vi "Prompt for File Path.vi"(0 "reference in":refnum<class "Generic Utilities.lvclass">, 5 "error in (no error)":errorcluster, 7 "Start Path":path, 9 "File Type":T1(ring)) -> (13 "selected path":path, 14 "reference out":refnum<class "Generic Utilities.lvclass">, 19 "error out":errorcluster)   [LabVIEW 2020, in "Generic Utilities.lvclass"]
uses:
  Generic Utilities.lvclass
  <vilib>/Utility/sysdir.llb/System Directory Type.ctl
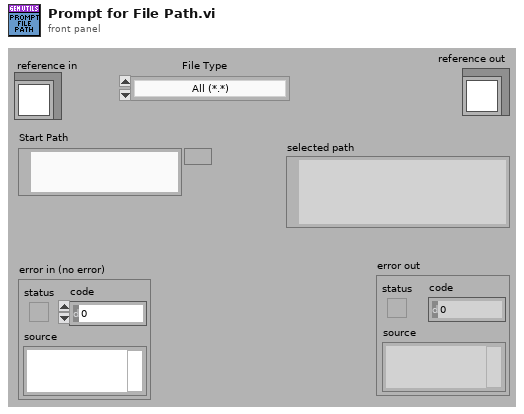
[diagram p1: front panel]
types:
  T1 = enum16{"All (*.*)", "Text (*.txt)", "Word (*.doc)", "Excel (*.xls)"}
  T2 = typedef "Generic Utilities.lvclass/ObjectAttributes.ctl" = cluster{"GUI Parameters":T3, "State Machine Control":cluster{"Timeout":i32, "State Queue":string[], "State History":string[], "State History Length":i32}, "Logging File Path":path, "OBJ not a refnum?":bool, "Timer Start":timestamp, "FP Refnums":T4}
  T3 = typedef "Generic Utilities.lvclass/GUI Parameters.ctl" = cluster{"Application Name":string, "GUI VI Ref":refnum<vi>, "Close Panel?":bool, "Message Window ref":refnum<vi>, "Version #":string}
  T4 = typedef "Generic Utilities.lvclass/FP Refnums.ctl" = cluster{"Panel refnum":refnum<vi>, "Control Labels":string[], "Refnums":refnum<vi>[]}
  T5 = typedef "System Directory Type.ctl" = i32
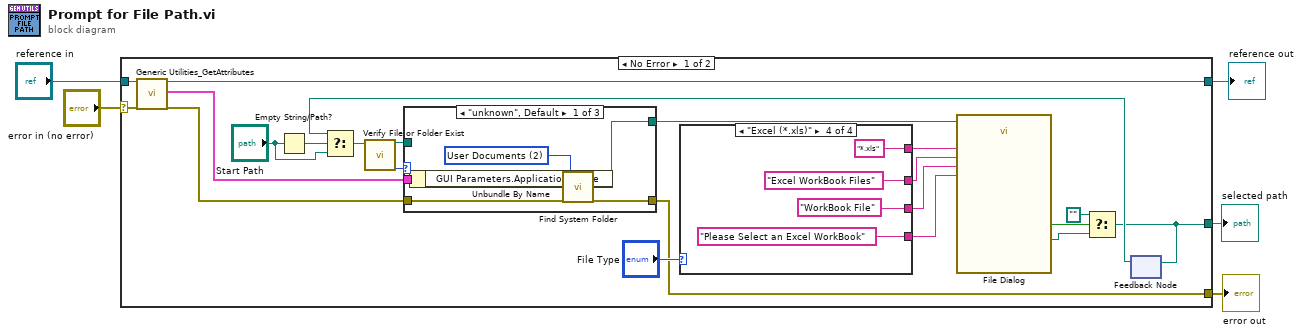
[diagram p0: block diagram]
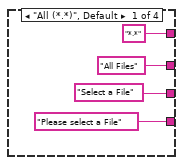
[diagram p2: hidden frame]
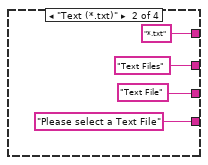
[diagram p3: hidden frame]
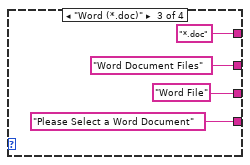
[diagram p4: hidden frame]
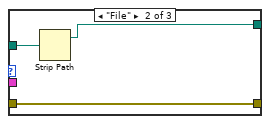
[diagram p5: hidden frame]
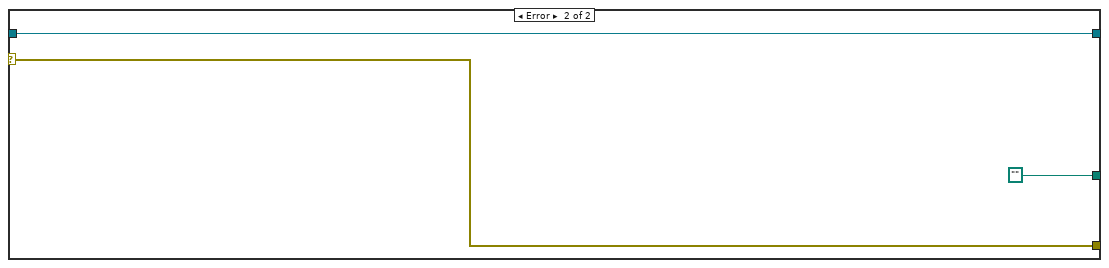
[diagram p7: hidden frame]
diagram:
  n1 = case shown="No Error" "error in (no error)" {
    selector: "error in (no error)" -> [w27 w57]
    tunnel: [w11 w57] -> w4
    tunnel: [w26 w56] -> w2
    tunnel: "reference in" -> [w24 w56]
    tunnel: [w7 path ""] -> w1
    frame No Error {
      n2 = call "Generic Utilities_GetAttributes.vi"("reference in"=w24, "error in (no error)"=w27) -> ("reference out"=w26:refnum<class "Generic Utilities.lvclass">, "attributes"=w25:T2, "error out"=w23:errorcluster)  [unwired: 14 in, 1 out]
      n3 = Empty String/Path?(string/path="Start Path") -> (empty?=w9:bool)
      n4 = case shown="\"Excel (*.xls)\"" "File Type" {
        tunnel: ["*.*" ("pattern (all files)") "*.txt" ("pattern (all files)") "*.doc" ("pattern (all files)") "*.xls" ("pattern (all files)")] -> w19
        tunnel: ["All Files" ("pattern label") "Text Files" ("pattern label") "Word Document Files" ("pattern label") "Excel WorkBook Files" ("pattern label")] -> w17
        tunnel: ["Select a File" ("button label") "Text File" ("button label") "Word File" ("button label") "WorkBook File" ("button label")] -> w16
        tunnel: ["Please select a File" ("button label") "Please select a Text File" ("button label") "Please Select a Word Document" ("button label") "Please Select an Excel WorkBook" ("button label")] -> w15
        frame "All (*.*)", Default {
        }
        frame "Text (*.txt)" {
        }
        frame "Word (*.doc)" {
        }
        frame "Excel (*.xls)" {
        }
      }
      n5 = feedback #1() -> (w10:path)  [unwired: 1 in]
      n6 = Select(t=w10, s=w9, f="Start Path") -> (s? t:f=w6:path)
      n7 = call "Verify File or Folder Exist.vi"("path"=w6) -> ("dup path"=w21:path, "Path Type"=w22:enum16{"unknown", "File", "Folder"})  [unwired: 16 in, 1 out]
      n8 = case shown="\"unknown\", Default" w22 {
        tunnel: w25 -> [w49 _ _]
        tunnel: w23 -> [w46 w50 w53]
        tunnel: [w44 w51 w54] -> w18
        tunnel: w21 -> [_ w52 w54]
        tunnel: [w45 w50 w53] -> w11
        frame "unknown", Default {
          w48 = T5 2 items=["User Home"=0, "User Desktop"=1, "User Documents"=2, "User Application Data"=3, "User Preferences"=4, "User Temporary"=5, "Public Documents"=6, "Public Application Data"=7, "Public Preferences"=8, "Public Cache"=13, "System Core Libraries"=9, "System Installed Libraries"=10, "Application Files"=11, "Boot Volume Root"=12] ("system directory type")
          n9 = Unbundle By Name(w49) -> ("GUI Parameters.Application Name"=w47:string)
          n10 = call "Find System Folder.vi"("Application Name"=w47, "error in (no error)"=w46, "system directory type"=w48) -> ("System Folder"=w44:path, "error out"=w45:errorcluster)  [unwired: 15 in]
        }
        frame "File" {
          n11 = Strip Path(path=w52) -> (stripped path=w51:path)  [unwired: 1 out]
        }
        frame "Folder" {
        }
      }
      n12 = call "File Dialog"("start path"=w18, "prompt"=w15, "button label"=w16, "pattern (all files)"=w19, "pattern label"=w17) -> ("selected path"=w13:path, "cancelled"=w14:bool)  [unwired: 7 in, 2 out]
      n13 = Select(t=path "", s=w14, f=w13) -> (s? t:f=w7:path)
      n14 = feedback-in #1(w7) -> ()
    }
    frame Error {
    }
  }
  "error out" <- w4
  "reference out" <- w2
  "selected path" <- w1
